vi "Engage Screwdriver.vi"(0 "reference in":refnum<class "SmartMotor.lvclass">, 2 "Range to Probe (Revolutions)":dbl=0.3, 4 "Number of Tries":i32=1, 5 "error in (no error)":errorcluster, 6 "UUT":refnum<class "UUT.lvclass">) -> (14 "reference out":refnum<class "SmartMotor.lvclass">, 18 "Screw Engaged":bool, 19 "error out":errorcluster)   [LabVIEW 2017, in "SmartMotor.lvclass"]
uses:
  SmartMotor.lvclass
  3-UUT/UUT_class/UUT.lvclass
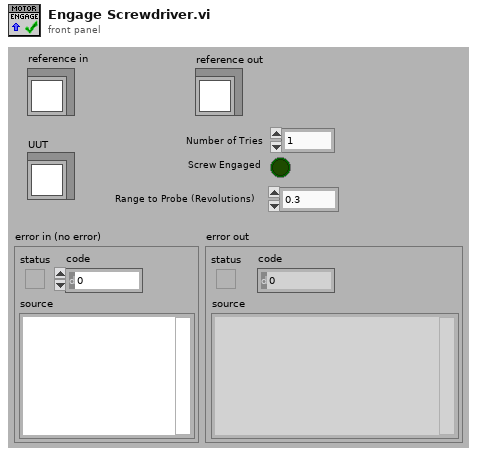
[diagram p1: front panel]
types:
  T1 = typedef "SmartMotor.lvclass/ObjectAttributes.ctl" = cluster{"SmartMotor Chain VISA Resource":refnum<visa-resource-name>, "SmartMotor Chain Address":i16, "Motor Absolute Position":i32, "Motor Relative Position":i32, "Motor Torque":i32, "Motor Voltage":i32, "Screwdriver Engaged":bool, "Screwdriver Torque Limit":i32, "Torque Monitor On/Off Status":bool, "Torque Monitor VI Reference":refnum<vi>, "Absolute Motor Torque (Filtered)":dbl, "SmartMotor Status":T2, "SmartMotor Error":T3}
  T2 = typedef "SmartMotor.lvclass/SmartMotor Status.ctl" = enum8{"Stopped", "Moving"}
  T3 = typedef "SmartMotor.lvclass/SmartMotor Error.ctl" = enum8{"None", "Read Error", "Low Voltage"}
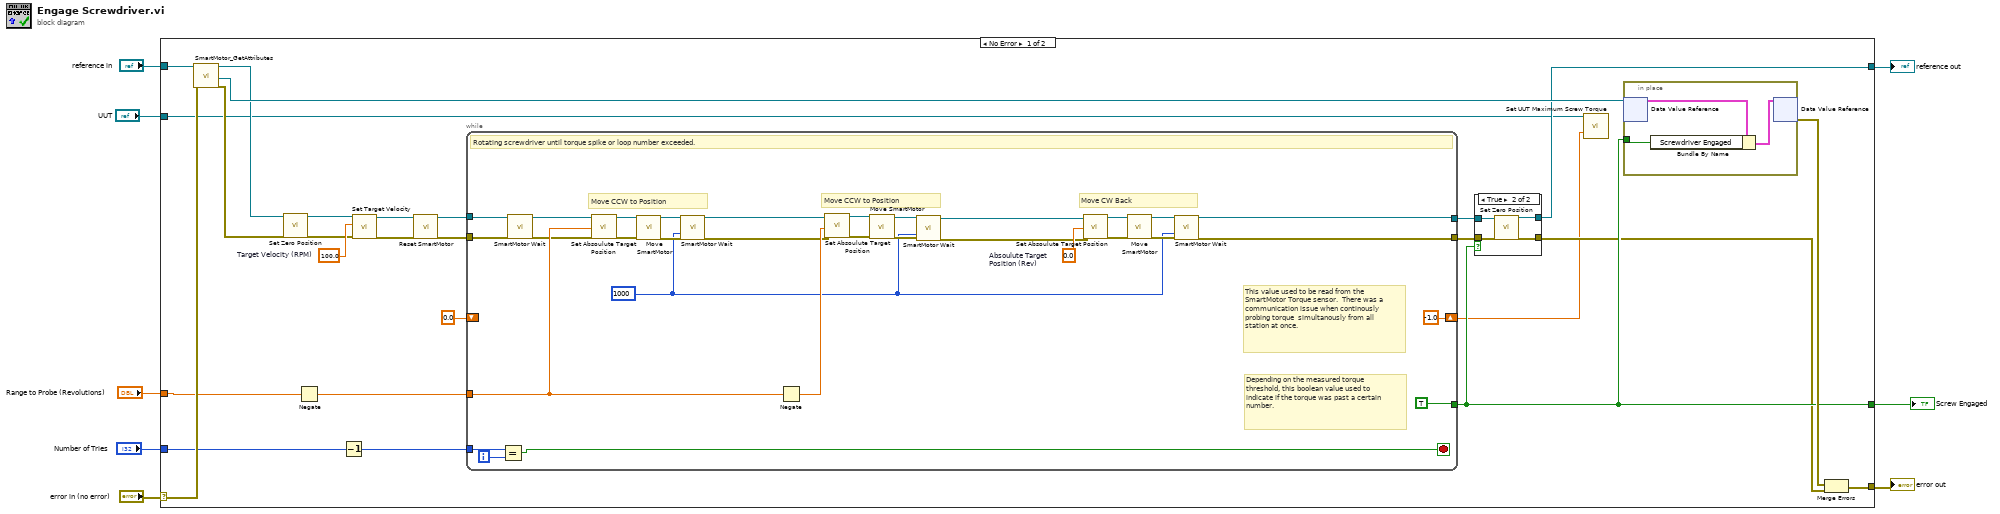
[diagram p0: block diagram]
diagram:
  n1 = case shown="No Error" "error in (no error)" {
    selector: "error in (no error)" -> [w33 w76]
    tunnel: [w31 w76] -> w7
    tunnel: [w20 w75] -> w5
    tunnel: "reference in" -> [w34 w75]
    tunnel: "Number of Tries" -> [w27 _]
    tunnel: [w26 _] -> w3
    tunnel: "Range to Probe (Revolutions)" -> [w18 _]
    tunnel: "UUT" -> [w17 _]
    frame No Error {
      w29 = 100.0  # Target Velocity (RPM)
      n2 = call "SmartMotor_GetAttributes.vi"("reference in"=w34, "error in (no error)"=w33) -> ("reference out"=w23:refnum<class "SmartMotor.lvclass">, "DataRef"=w30:refnum<data-value>, "error out"=w22:errorcluster)  [unwired: 14 in, 1 out]
      n3 = call-dynamic "Set Zero Position.vi"("reference in"=w23, "error in (no error)"=w22) -> ("reference out"=w24:refnum<class "SmartMotor.lvclass">, "error out"=w21:errorcluster)  [unwired: 16 in]
      n4 = Negate(x=w18) -> (-x=w19:dbl)
      n5 = Decrement(x=w27) -> (x-1=w28:i32)
      n6 = call-dynamic "Set Target Velocity.vi"("reference in"=w24, "Target Velocity (RPM)"=w29, "error in (no error)"=w21) -> ("reference out"=w12:refnum<class "SmartMotor.lvclass">, "error out"=w11:errorcluster)  [unwired: 15 in]
      n7 = call-dynamic "Reset SmartMotor.vi"("reference in"=w12, "error in (no error)"=w11) -> ("reference out"=w10:refnum<class "SmartMotor.lvclass">, "error out"=w9:errorcluster)  [unwired: 16 in]
      n8 = while {
        tunnel: [w36] -> w25
        tunnel: [TRUE] -> w26
        tunnel: w28 -> [w59]
        tunnel: w19 -> [w55]
        shift-right: [-1.0] -> w14
        shift-left: 0.0 -> [_]
        tunnel: [w37] -> w13
        tunnel: w10 -> [w53]
        tunnel: w9 -> [w51]
        i -> [w60]
        stop <- w58 stop-if-true
        w35 = u32 1000 ("Number of Milliseconds to Wait")
        w61 = 0.0  # Absoulute Target  Position (Rev)
        # "Depending on the measured torque threshold, this boolean value used to indicate if the torque was past a certain number."
        # "This value used to be read from the SmartMotor Torque sensor.  There was a communication issue when continously probing torque  simultanously from all station at once."
        # "Move CCW to Position"
        # "Move CW Back"
        # "Move CCW to Position"
        # "Rotating screwdriver until torque spike or loop number exceeded."
        n9 = Equal?(x=w59, y=w60) -> (x = y?=w58:bool)
        n10 = call-dynamic "SmartMotor Wait.vi"("reference in"=w53, "error in (no error)"=w51) -> ("reference out"=w52:refnum<class "SmartMotor.lvclass">, "error out"=w50:errorcluster)  [unwired: 16 in]
        n11 = call-dynamic "Set Absoulute Target Position.vi"("reference in"=w52, "Absoulute Target Position (Revolutions)"=w55, "error in (no error)"=w50) -> ("reference out"=w63:refnum<class "SmartMotor.lvclass">, "error out"=w62:errorcluster)  [unwired: 15 in]
        n12 = call-dynamic "Move SmartMotor.vi"("reference in"=w63, "error in (no error)"=w62) -> ("reference out"=w47:refnum<class "SmartMotor.lvclass">, "error out"=w45:errorcluster)  [unwired: 16 in]
        n13 = call-dynamic "SmartMotor Wait.vi"("reference in"=w47, "Number of Milliseconds to Wait"=w35, "error in (no error)"=w45) -> ("reference out"=w46:refnum<class "SmartMotor.lvclass">, "error out"=w44:errorcluster)  [unwired: 15 in]
        n14 = Negate(x=w55) -> (-x=w54:dbl)
        n15 = call-dynamic "Set Absoulute Target Position.vi"("reference in"=w46, "Absoulute Target Position (Revolutions)"=w54, "error in (no error)"=w44) -> ("reference out"=w57:refnum<class "SmartMotor.lvclass">, "error out"=w56:errorcluster)  [unwired: 15 in]
        n16 = call-dynamic "Move SmartMotor.vi"("reference in"=w57, "error in (no error)"=w56) -> ("reference out"=w43:refnum<class "SmartMotor.lvclass">, "error out"=w42:errorcluster)  [unwired: 16 in]
        n17 = call-dynamic "SmartMotor Wait.vi"("reference in"=w43, "Number of Milliseconds to Wait"=w35, "error in (no error)"=w42) -> ("reference out"=w41:refnum<class "SmartMotor.lvclass">, "error out"=w40:errorcluster)  [unwired: 15 in]
        n18 = call-dynamic "Set Absoulute Target Position.vi"("reference in"=w41, "Absoulute Target Position (Revolutions)"=w61, "error in (no error)"=w40) -> ("reference out"=w65:refnum<class "SmartMotor.lvclass">, "error out"=w64:errorcluster)  [unwired: 15 in]
        n19 = call-dynamic "Move SmartMotor.vi"("reference in"=w65, "error in (no error)"=w64) -> ("reference out"=w39:refnum<class "SmartMotor.lvclass">, "error out"=w38:errorcluster)  [unwired: 16 in]
        n20 = call-dynamic "SmartMotor Wait.vi"("reference in"=w39, "Number of Milliseconds to Wait"=w35, "error in (no error)"=w38) -> ("reference out"=w37:refnum<class "SmartMotor.lvclass">, "error out"=w36:errorcluster)  [unwired: 15 in]
      }
      n21 = case shown="True" w26 {
        tunnel: w25 -> [w67 w71]
        tunnel: [w67 w70] -> w16
        tunnel: [w66 w69] -> w20
        tunnel: w13 -> [w66 w68]
        frame False {
        }
        frame True {
          n22 = call-dynamic "Set Zero Position.vi"("reference in"=w68, "error in (no error)"=w71) -> ("reference out"=w69:refnum<class "SmartMotor.lvclass">, "error out"=w70:errorcluster)  [unwired: 16 in]
        }
      }
      n23 = call-dynamic "Set UUT Maximum Screw Torque.vi"("reference in"=w17, "Maximum Screw Torque"=w14) -> ()  [unwired: 16 in, 2 out]
      n24 = in-place {
        in-place-border: w26 -> [w72]
        n25 = in-place-dvr #1(w30) -> (w74:T1)  [unwired: 1 out]
        n26 = Bundle By Name(cluster=w74, "Screwdriver Engaged"=w72) -> (w73:T1)
        n27 = in-place-dvr #1(w73) -> (w32:errorcluster)  [unwired: 1 out]
      }
      n28 = Merge Errors(w32, w16) -> (w31:errorcluster)
    }
    frame Error {
    }
  }
  "error out" <- w7
  "reference out" <- w5
  "Screw Engaged" <- w3
